vi "Init Events.vi"(8 "error in (no error)":errorcluster, 11 "SB App in":refnum<class "SB App.lvclass">) -> (0 "error out":errorcluster, 3 "SB App out":refnum<class "SB App.lvclass">)   [LabVIEW 2020, in "SB App.lvlib" / "SB App.lvclass"]
uses:
  SB App.lvclass
  Board Size Update.ctl
  Game Start Data.ctl
  SquareBattle/Team Start Info.ctl
  SquareBattle/Team/Team.lvclass
  SquareBattle/Position.ctl
  Start Position Data.ctl
  SquareBattle/Team ID.ctl
  SB App.lvclass/SB App.ctl
  SB App.lvlib
  SquareBattle/SquareBattle.lvlib
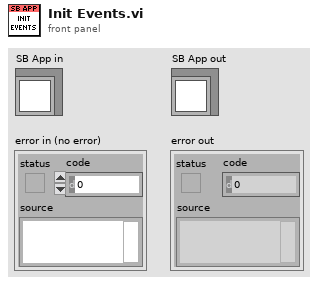
[diagram p1: front panel]
types:
  T1 = typedef "SB App.lvlib/Start Position Data.ctl" = cluster{"Team ID":T2, "Position":T3}
  T2 = typedef "SquareBattle.lvlib/Team ID.ctl" = u32
  T3 = typedef "SquareBattle.lvlib/Position.ctl" = cluster{"Row":i32, "Col":i32}
  T4 = typedef "SB App.lvlib/Game Start Data.ctl" = cluster{"Team Starts":T5[], "Board Size":i32, "Replication Rounds":u32}
  T5 = typedef "SquareBattle.lvlib/Team Start Info.ctl" = cluster{"Team":refnum<class "Team.lvclass">, "Position":T3}
  T6 = typedef "SB App.lvlib/Board Size Update.ctl" = cluster{"Board Size":i32}
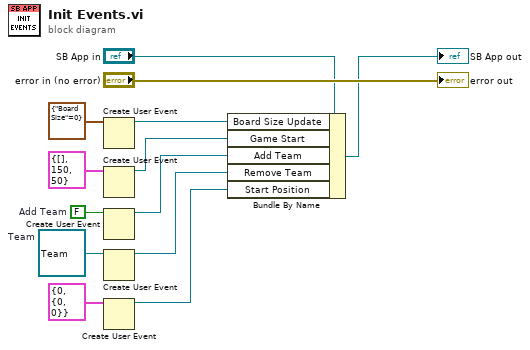
[diagram p0: block diagram]
diagram:
  w4 = refnum<class "Team.lvclass"> refnum  # Team
  w6 = FALSE  # Add Team
  n1 = Create User Event(user event datatype=T6 {"Board Size"=0} ("Board Size Update")) -> (user event=w9:refnum<user-event>)  [unwired: 1 in, 1 out]
  n2 = Create User Event(user event datatype=T4 {"Team Starts"=[], "Board Size"=150, "Replication Rounds"=50} ("Game Start Data")) -> (user event=w7:refnum<user-event>)  [unwired: 1 in, 1 out]
  n3 = Create User Event(user event datatype=w6) -> (user event=w5:refnum<user-event>)  [unwired: 1 in, 1 out]
  n4 = Create User Event(user event datatype=w4) -> (user event=w3:refnum<user-event>)  [unwired: 1 in, 1 out]
  n5 = Create User Event(user event datatype=T1 {"Team ID"=0, "Position"={"Row"=0, "Col"=0}} ("Start Position Data")) -> (user event=w1:refnum<user-event>)  [unwired: 1 in, 1 out]
  n6 = Bundle By Name(cluster="SB App in", "Board Size Update"=w9, "Game Start"=w7, "Add Team"=w5, "Remove Team"=w3, "Start Position"=w1) -> (→"SB App out":refnum<class "SB App.lvclass">)
  "error out" <- "error in (no error)"
